vi "Coord window-Best match.vi"(9 "Values to compare with the target":dbl[](array[numeric]), 11 "Target value":dbl) -> (1 "Indexes of matching elements":i32[](array[numeric]))   [LabVIEW 2017]
uses:
  Global Variables/gl_UI Ctrl Refs.vi
panel:
  out "Could not detect":bool
  in  "Maximum filter window in FOV":sgl=2.0
  in  "Filter window width increment (um)":dbl=100.0
  # "<---Can be further optimised"
  # "<---Can be further optimised"
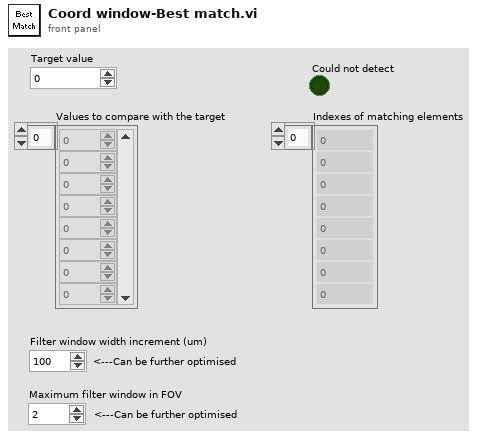
[diagram p1: front panel]
types:
  T1 = typedef "UI ctrl refs cluster.ctl" = cluster{"Top level VI path":path, "Top level VI ref":refnum<vi>, "User menu ref":refnum<k9>, "Sub Panel control":refnum<vi>, "Imaging Param Tab":refnum<vi>, "Occurrence-Start drivers":refnum<k4>, "Occurrence-Speed logging initialised":refnum<k4>, "Occurrence-XYZ stage initialised":refnum<k4>, "Exit button":refnum<vi>, "Status ind":refnum<vi>, "Set as origin":refnum<vi>, "Speed Logging":refnum<vi>, "Time Lapse":refnum<vi>, "Live Imaging":refnum<vi>, "AOL Z Stack":refnum<vi>, "Motor Z Stack":refnum<vi>, "Funct Acq button":refnum<vi>, "Hard Shutter":refnum<vi>, "Virtual Shutter":refnum<vi>, "Laser Power":refnum<vi>, "AOL Mode":refnum<vi>, "Frame Size":refnum<vi>, "Field of View":refnum<vi>, "Dwell Time":refnum<vi>, "Zoom":refnum<vi>, "AOL Z":refnum<vi>, "Objective":refnum<vi>, "Axis":refnum<vi>, "Paths & Names":refnum<vi>, "Experiment folder path (ind.)":refnum<vi>, "Last State (Ind.)":refnum<vi>, "Laser wavelength ind (nm)":refnum<vi>, "Averages":refnum<vi>, "Angle (degrees)":refnum<vi>, "X centre":refnum<vi>, "Y centre":refnum<vi>, "Plane Mode":refnum<vi>, "# Planes":refnum<vi>, "Z Start":refnum<vi>, "Z Stop":refnum<vi>, "Z Step":refnum<vi>, "PMT 1":refnum<vi>, "PMT 2":refnum<vi>, "Stage XYZ Position":refnum<vi>, "Pockels@Z Start":refnum<vi>, "Pockels@Z Stop":refnum<vi>, "Obtain Z Start":refnum<vi>, "Obtain Z Stop":refnum<vi>, "Live stim.trig.period":refnum<vi>, "Live stim.trig.enable":refnum<vi>, "Movement Correction":refnum<vi>, "Load Reference Image":refnum<vi>, "XY Stage Move":refnum<vi>, "MovCor Cluster":refnum<vi>, "RefDAQParam":refnum<vi>, "Funct. Acq. Pockels Modulation":refnum<vi>, "Background MovCor":refnum<vi>, "Ref Laser Power":refnum<vi>, "Enable Video Recording":refnum<vi>, "Video Record-Live Imaging":refnum<vi>, "Video Record-Funct acq":refnum<vi>, "Reference Source":refnum<vi>, "AOL Z-stack Chirps Ready (ind)":refnum<vi>, "Target time between mov.cor. ref triggers (ms)":refnum<vi>, "Funct. Acq. Ref frame save":refnum<vi>, "Tracking button":refnum<vi>, "Show ref plots window":refnum<vi>, "Center freq ind (nm)":refnum<vi>, "Pickup mode (ind)":refnum<vi>, "Logging queue (ind)":refnum<vi>, "Back aperture power (ind.)":refnum<vi>, "Power after objective (ind.)":refnum<vi>, "Switch user":refnum<vi>}
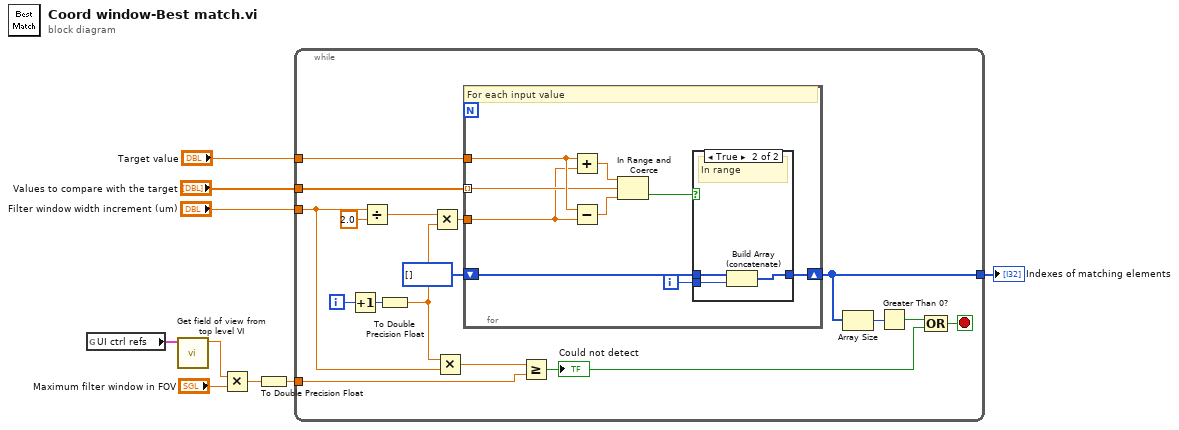
[diagram p0: block diagram]
diagram:
  n1 = global read "gl_UI Ctrl Refs.vi" "UI ctrl refs"() -> (w7:T1)
  n2 = call "Get field of view from top level VI.vi"("UI ctrl refs"=w7) -> ("Field of view (um)"=w3:sgl)  [unwired: 10 in]
  n3 = Multiply(x=w3, y="Maximum filter window in FOV") -> (x*y=w2:sgl)
  n4 = To Double Precision Float(number=w2) -> (double precision float=w5:dbl)
  n5 = while {
    tunnel: "Target value" -> [w25]
    tunnel: "Values to compare with the target" -> [w24]
    tunnel: w5 -> [w21]
    tunnel: [w17] -> w6
    tunnel: "Filter window width increment (um)" -> [w10]
    i -> [w26]
    stop <- w18 stop-if-true
    n6 = Increment(x=w26) -> (x+1=w16:i32)
    n7 = Divide(x=w10, y=2.0) -> (x/y=w12:dbl)
    n8 = To Double Precision Float(number=w16) -> (double precision float=w11:dbl)
    n9 = Multiply(x=w12, y=w11) -> (x*y=w14:dbl)
    n10 = Multiply(x=w11, y=w10) -> (x*y=w15:dbl)
    n11 = for {
      tunnel: w25 -> [w34]
      tunnel: w24 -> [w32] mode=indexing
      shift-right: [w29] -> w17
      shift-left: i32[] [] -> [w28]
      tunnel: w14 -> [w27]
      i -> [w30]
      # "For each input value"
      n12 = Add(x=w34, y=w27) -> (x+y=w35:dbl)
      n13 = Subtract(x=w34, y=w27) -> (x-y=w33:dbl)
      n14 = In Range and Coerce(upper limit=w35, x=w32, lower limit=w33) -> (In Range?=w31:bool)  [unwired: 1 out]
      n15 = case shown="True" w31 {
        tunnel: w30 -> [_ w39]
        tunnel: [w36 w38] -> w29
        tunnel: w28 -> [w36 w37]
        frame False {
          # "OOR"
        }
        frame True {
          # "In range"
          n16 = Build Array (concatenate)(w37, w39) -> (w38:i32[])
        }
      }
    }
    n17 = Greater Or Equal?(x=w15, y=w21) -> (x >= y?=w19:bool)
    "Could not detect" <- w19
    n18 = Array Size(array=w17) -> (size(s)=w22:i32)
    n19 = Greater Than 0?(x=w22) -> (x > 0?=w20:bool)
    n20 = Compound Arithmetic op=OR(w20, w19) -> (w18:bool)
  }
  "Indexes of matching elements" <- w6
